vi "LibraryInit.vi"(9 "error in (no error)":errorcluster) -> (0 "error out":errorcluster, 3 "Library Initialized":bool)   [LabVIEW 2015]
uses:
  XGL_DPP.lvlib
panel:
  out "Error code":i32
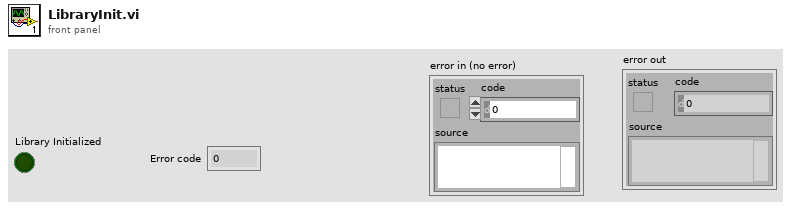
[diagram p1: front panel]
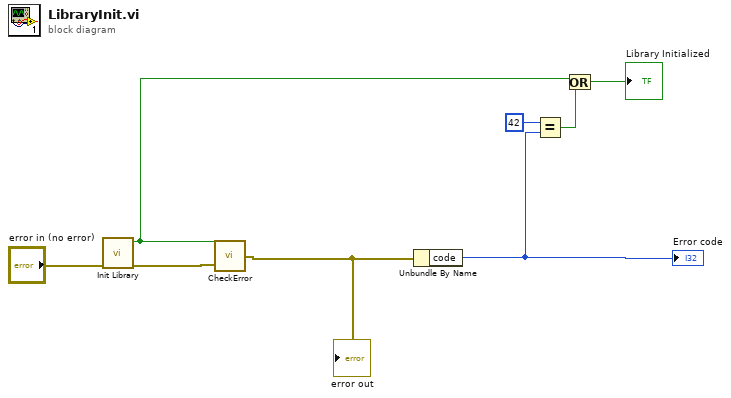
[diagram p0: block diagram]
diagram:
  n1 = call "Init Library.vi"("error in (no error)"="error in (no error)") -> ("error out"=w7:errorcluster, "function return"=w1:bool)  [unwired: 9 in]
  n2 = call "CheckError.vi"("error in (no error)"=w7, "ret_val"=w1) -> ("error out"=w8:errorcluster)
  "error out" <- w8
  n3 = Unbundle By Name(w8) -> ("code"=w3:i32)
  "Error code" <- w3
  n4 = Equal?(x=42, y=w3) -> (x = y?=w4:bool)
  n5 = Or(x=w1, y=w4) -> (x .or. y?=→"Library Initialized":bool)
